vi "UploadResultToSystemlink.vi"() -> ()   [LabVIEW 2018]
uses:
  Execution/TestMonitor.lvclass
  Report Information/DUT Information.ctl
  Report Information/Station Information.ctl
  Report Information/Test Information.ctl
  Result/Result.lvclass
  Step/Execution/Step Status.ctl
  Report Information/Report Information.lvclass
  Step/Execution/Step.lvclass
panel:
  out "error out":errorcluster
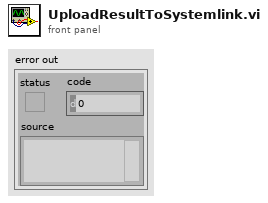
[diagram p1: front panel]
types:
  T1 = typedef "Step.lvclass/Step Status.ctl" = enum16{"Start", "Passed", "Failed", "Error", "Done", "Terminated", "Skipped", "Running"}
  T2 = typedef "Report Information.lvclass/Test Information.ctl" = cluster{"UUT Result":string, "Sequence Name":string, "Sequence Version":string}
  T3 = typedef "Report Information.lvclass/Station Information.ctl" = cluster{"Station ID":string, "Station Serial Number":string}
  T4 = typedef "Report Information.lvclass/DUT Information.ctl" = cluster{"DUT Serial Number":string, "DUT Info":string}
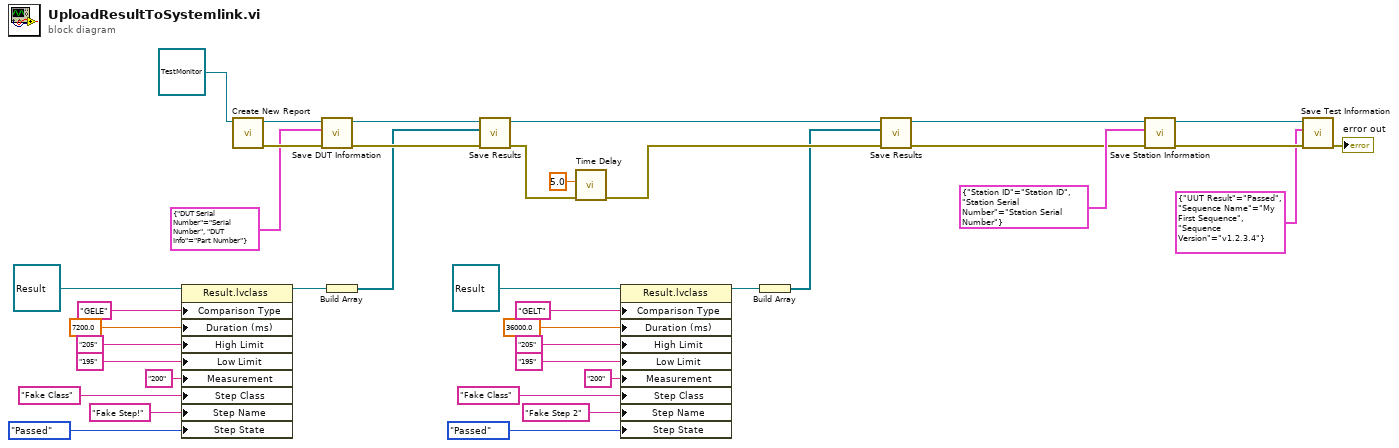
[diagram p0: block diagram]
diagram:
  n1 = property class="Result.lvclass"(reference=refnum<class "Result.lvclass"> refnum ("Result.lvclass"), "Comparison Type"="GELE", "Duration (ms)"=7200.0, "High Limit"="205", "Low Limit"="195", "Measurement"="200", "Step Class"="Fake Class", "Step Name"="Fake Step!", "Step State"=Step_Status."Passed") -> (reference out=w21:refnum<class "Result.lvclass">)  [unwired: 1 in, 1 out]
  n2 = call-dynamic "Create New Report.vi"("TestMonitor in"=refnum<class "TestMonitor.lvclass"> refnum ("TestMonitor.lvclass")) -> ("error out"=w32:errorcluster, "TestMonitor out"=w38:refnum<class "TestMonitor.lvclass">)  [unwired: 9 in]
  n3 = call-dynamic "Save DUT Information.vi"("error in (no error)"=w32, "DUT Info"=T4 {"DUT Serial Number"="Serial Number", "DUT Info"="Part Number"}, "TestMonitor in"=w38) -> ("error out"=w33:errorcluster, "TestMonitor out"=w37:refnum<class "TestMonitor.lvclass">)  [unwired: 7 in]
  n4 = Build Array(w21) -> (w20:refnum<class "Result.lvclass">[])
  n5 = call-dynamic "Save Results.vi"("error in (no error)"=w33, "Results"=w20, "TestMonitor in"=w37) -> ("error out"=w34:errorcluster, "TestMonitor out"=w3:refnum<class "TestMonitor.lvclass">)  [unwired: 7 in]
  n6 = call "Time Delay"("error in (no error)"=w34, "Delay Time (s)"=5.0) -> ("error out"=w16:errorcluster)  [unwired: 9 in]
  n7 = property class="Result.lvclass"(reference=refnum<class "Result.lvclass"> refnum ("Result.lvclass"), "Comparison Type"="GELT", "Duration (ms)"=36000.0, "High Limit"="205", "Low Limit"="195", "Measurement"="200", "Step Class"="Fake Class", "Step Name"="Fake Step 2", "Step State"=Step_Status."Passed") -> (reference out=w14:refnum<class "Result.lvclass">)  [unwired: 1 in, 1 out]
  n8 = Build Array(w14) -> (w4:refnum<class "Result.lvclass">[])
  n9 = call-dynamic "Save Results.vi"("error in (no error)"=w16, "Results"=w4, "TestMonitor in"=w3) -> ("error out"=w15:errorcluster, "TestMonitor out"=w2:refnum<class "TestMonitor.lvclass">)  [unwired: 7 in]
  n10 = call-dynamic "Save Station Information.vi"("error in (no error)"=w15, "Station Info"=T3 {"Station ID"="Station ID", "Station Serial Number"="Station Serial Number"}, "TestMonitor in"=w2) -> ("error out"=w35:errorcluster, "TestMonitor out"=w36:refnum<class "TestMonitor.lvclass">)  [unwired: 7 in]
  n11 = call-dynamic "Save Test Information.vi"("error in (no error)"=w35, "Test Information"=T2 {"UUT Result"="Passed", "Sequence Name"="My First Sequence", "Sequence Version"="v1.2.3.4"}, "TestMonitor in"=w36) -> ("error out"=→"error out":errorcluster)  [unwired: 7 in, 1 out]
